vi "setLevel.vi"(8 "error in (no error)":errorcluster, 10 "Level":u8, 11 "Change Level in":refnum<class "Change Level.lvclass">) -> (0 "error out":errorcluster, 3 "Change Level out":refnum<class "Change Level.lvclass">)   [LabVIEW 2019, in "Change Level.lvclass"]
uses:
  Change Level.lvclass
  Change Level.lvclass/Change Level.ctl
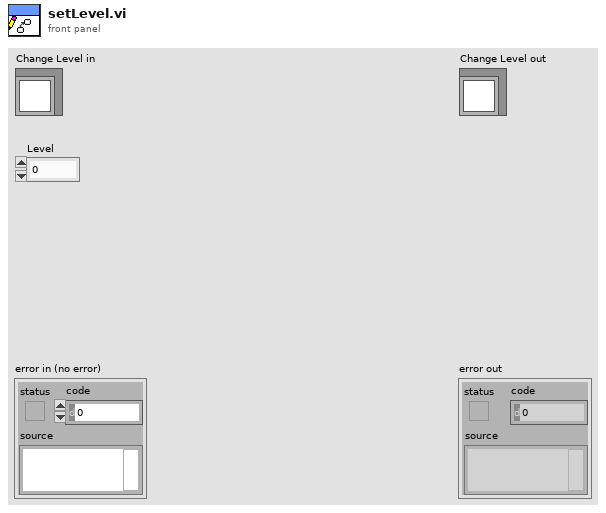
[diagram p1: front panel]
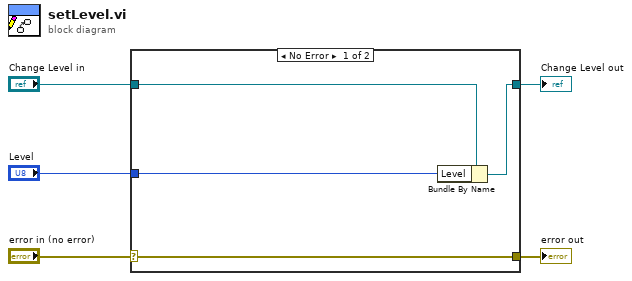
[diagram p0: block diagram]
diagram:
  n1 = case shown="No Error" "error in (no error)" {
    selector: "error in (no error)" -> [w9 w10]
    tunnel: [w9 w10] -> w4
    tunnel: [w7 w11] -> w2
    tunnel: "Change Level in" -> [w8 w11]
    tunnel: "Level" -> [w6 _]
    frame No Error {
      n2 = Bundle By Name(cluster=w8, "Level"=w6) -> (w7:refnum<class "Change Level.lvclass">)
    }
    frame Error {
    }
  }
  "error out" <- w4
  "Change Level out" <- w2
